vi "Lavatory_System..vi"(11 "Error_In":errorcluster) -> (15 "Error_Out":errorcluster)   [LabVIEW 2021]
doc: "This is the Main VI that performs the Lavatory system."
uses:
  Controls/Lavatory.ctl
  Controls/Lavatory_Data.ctl
  Controls/Queue_Operation_Select.ctl
  Controls/Timer_Operation_Select.ctl
panel:
  in  "Stop_Simulation":bool
  in  "Alarm_Timer_Limit":dbl=2.0 caption="Alarm Timer Limit" min=1.0 max=300.0
  out "Alarm_Timer_D":dbl caption="Alarm Timer D"
  out "Alarm_Timer_C":dbl caption="Alarm Timer C"
  in  "Lavatory_D_Occupied":bool caption="Lavatory D Occupied"
  in  "Lavatory_C_Occupied":bool caption="Lavatory C Occupied"
  out "Alarm_Timer_B":dbl caption="Alarm Timer B"
  out "Alarm_Timer_A":dbl caption="Alarm Timer A"
  in  "Lavatory_B_Occupied":bool caption="Lavatory B Occupied"
  in  "Lavatory_A_Occupied":bool caption="Lavatory A Occupied"
  out "Rear_Lavatories_Occupied":bool caption="Lavatories\nOccupied"
  out "Front_Lavatories_Occupied":bool caption="Lavatories\nOccupied"
  in  "Alarm_Achnowledge":bool caption="Alarm Achnowledge"
  out "Lavatory":string
  out "Alarm":bool
  in  "Seatbelt_Sign_ON":bool caption="Seatbelt Sign ON"
  out "Lavatory_A":T1 caption="Lavatory A"
  out "Lavatory_B":T1 caption="Lavatory B"
  out "Lavatory_D":T1 caption="Lavatory D"
  out "Lavatory_C":T1 caption="Lavatory C"
  # "Airplane Lavatory Signs"
  # "Front"
  # "Rear"
  # "Steward's Area"
  # "Simulation Contols & Indicators"
  # "Secs"
  # "Secs"
  # "Secs"
  # "Secs"
  # "Secs"
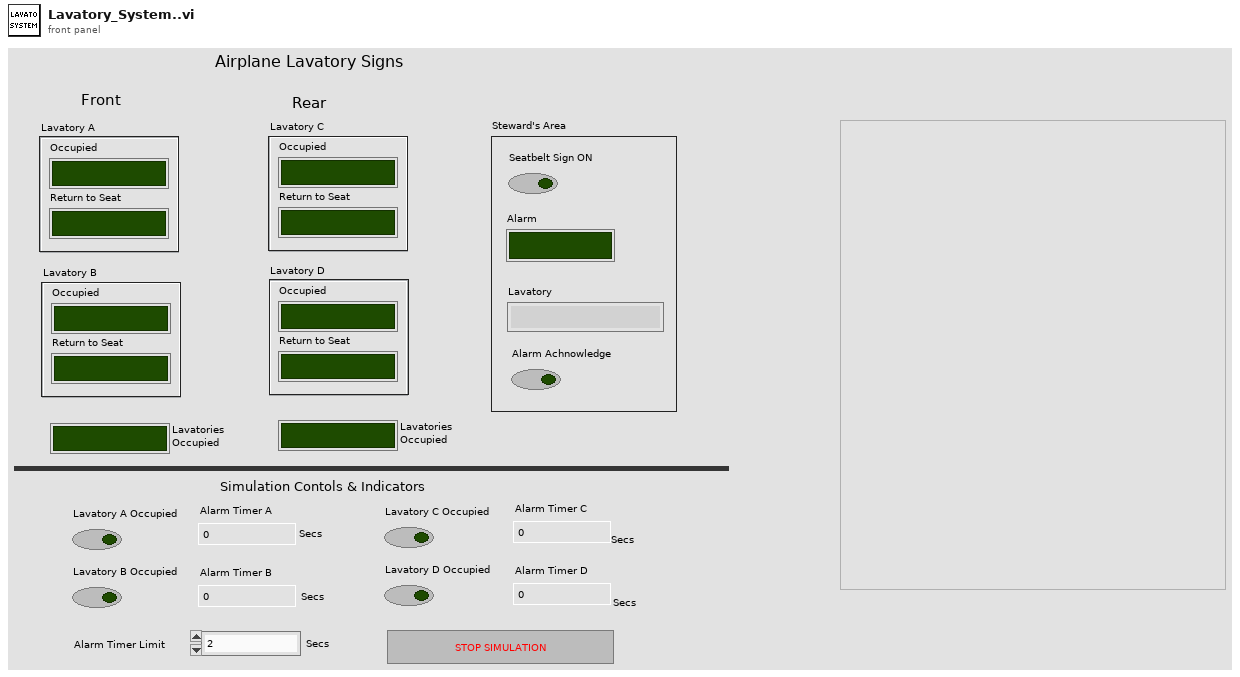
[diagram p1: front panel]
types:
  T1 = typedef "Lavatory.ctl" = cluster{"Occupied":bool, "Return_To_Seat":bool}
  T2 = typedef "Queue_Operation_Select.ctl" = enum16{"Obtain_Queue", "Enqueue", "Enqueue_N", "Enqueue_at_End", "Dequeue", "Flush", "Release_Queue"}
  T3 = typedef "Lavatory_Data.ctl" = cluster{"Lavatory":T1, "Lavatory_Name":string[], "Rear_Lavatories_Occupied":bool, "Front_Lavatories_Occupied":bool, "Alarm_Time":dbl[], "Alarm":bool, "Alarm_Message":string, "Alarm_Timer_Limit":dbl, "Seatbelt_Sign_ON":bool, "Occupied":bool[], "Return_To_Seat_F":bool[], "Lavatory_Reference":refnum<vi>[], "Time_Out?":bool[], "Lavatory_Controls":refnum<vi>[]}
  T4 = typedef "Timer_Operation_Select.ctl" = enum16{"Initialize", "Start_Timer", "Time_Out?", "Stop_Timer"}
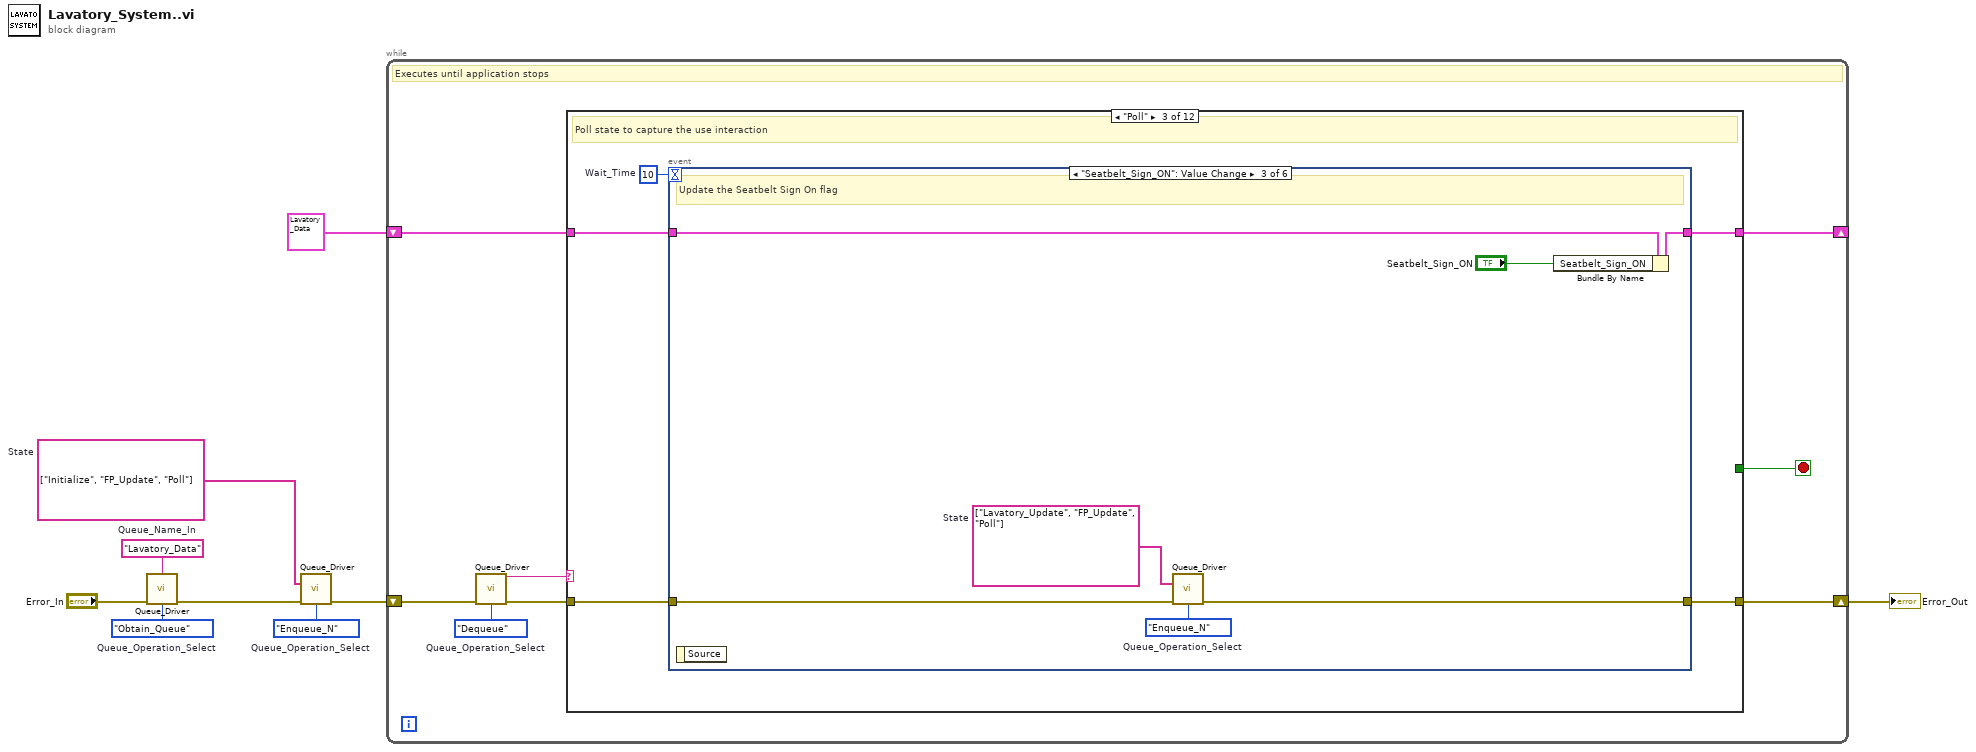
[diagram p0: block diagram]
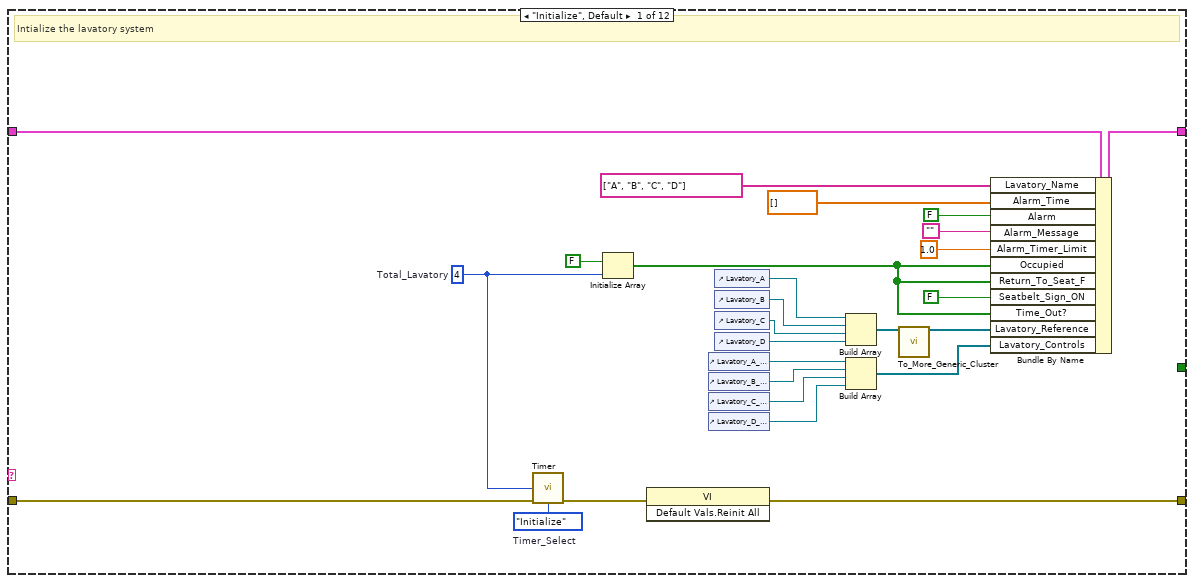
[diagram p2: hidden frame]
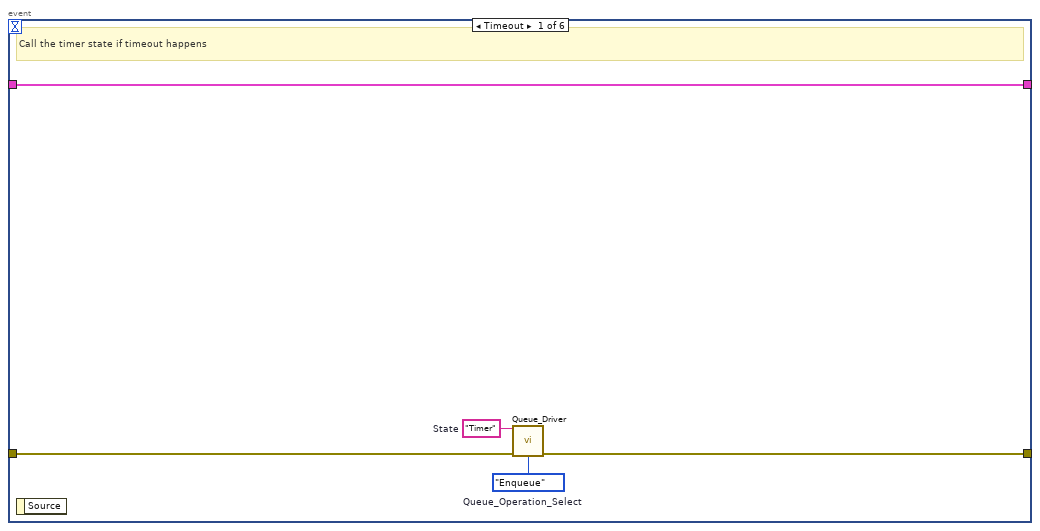
[diagram p4: hidden frame]
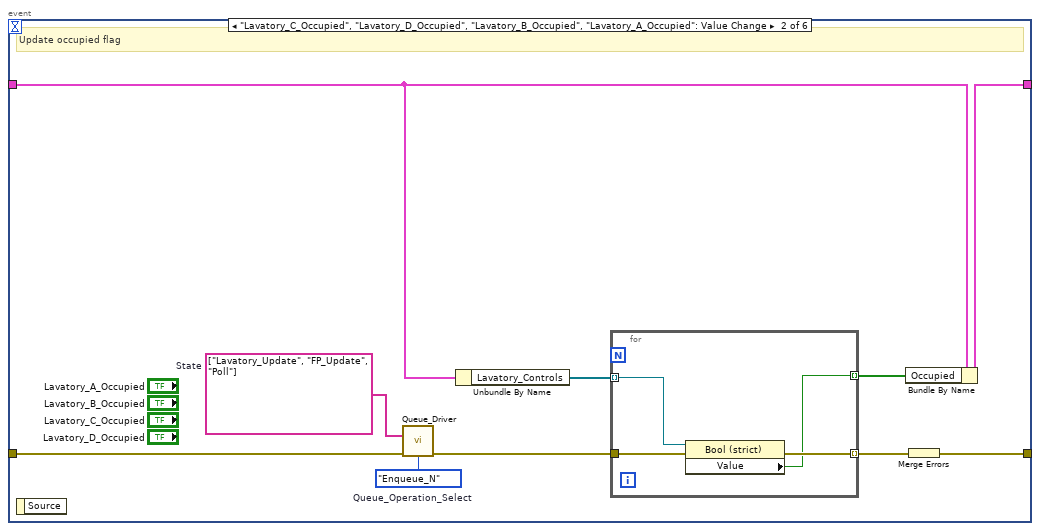
[diagram p5: hidden frame]
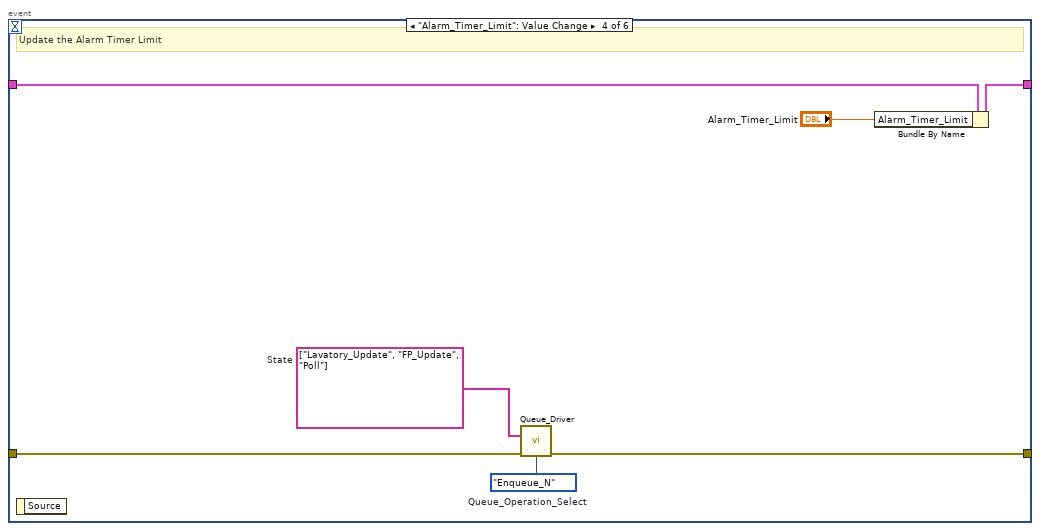
[diagram p6: hidden frame]
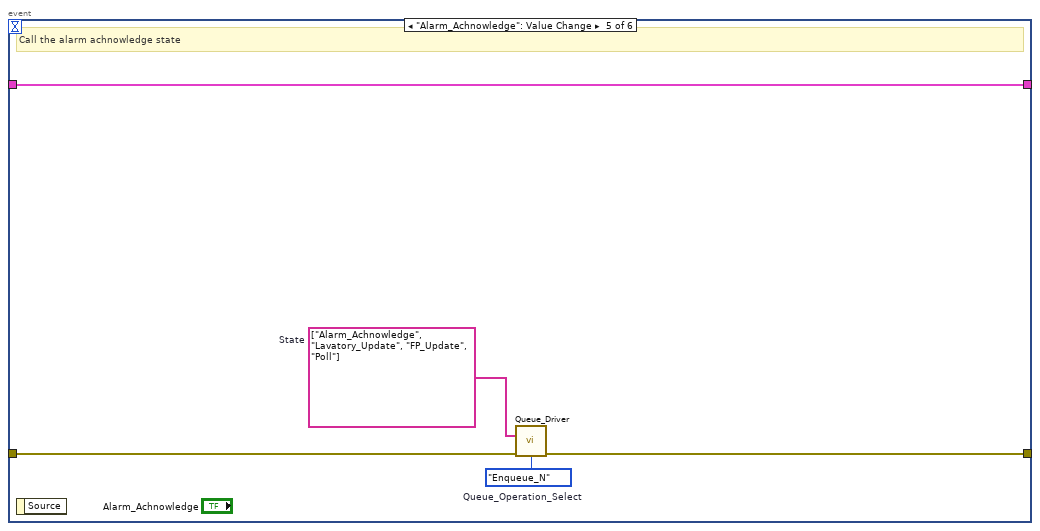
[diagram p7: hidden frame]
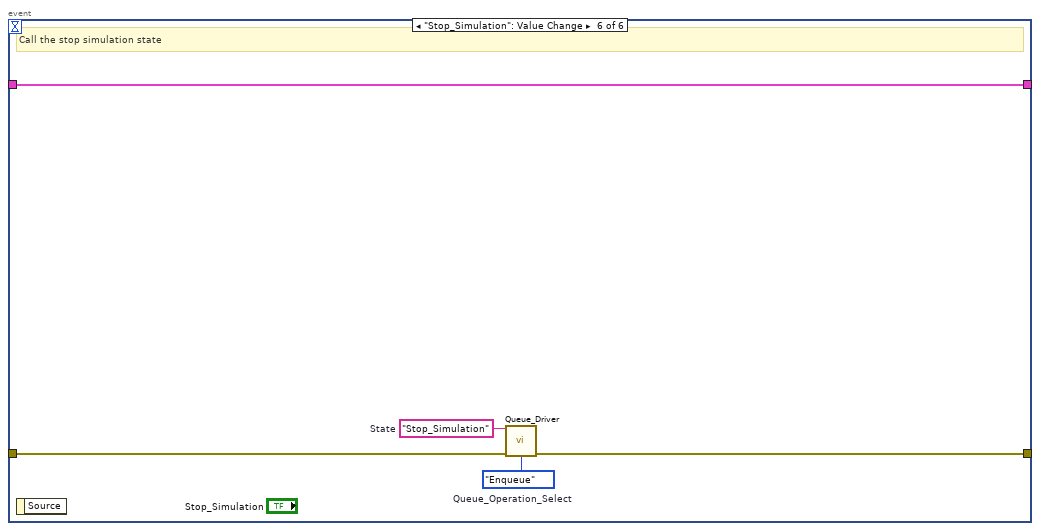
[diagram p8: hidden frame]
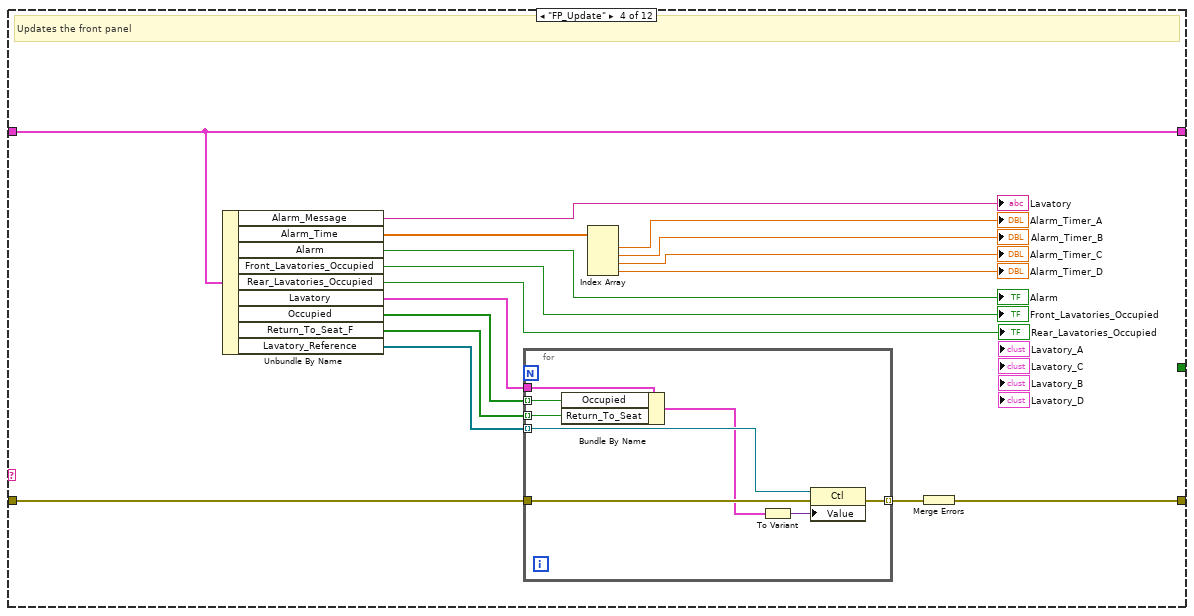
[diagram p9: hidden frame]
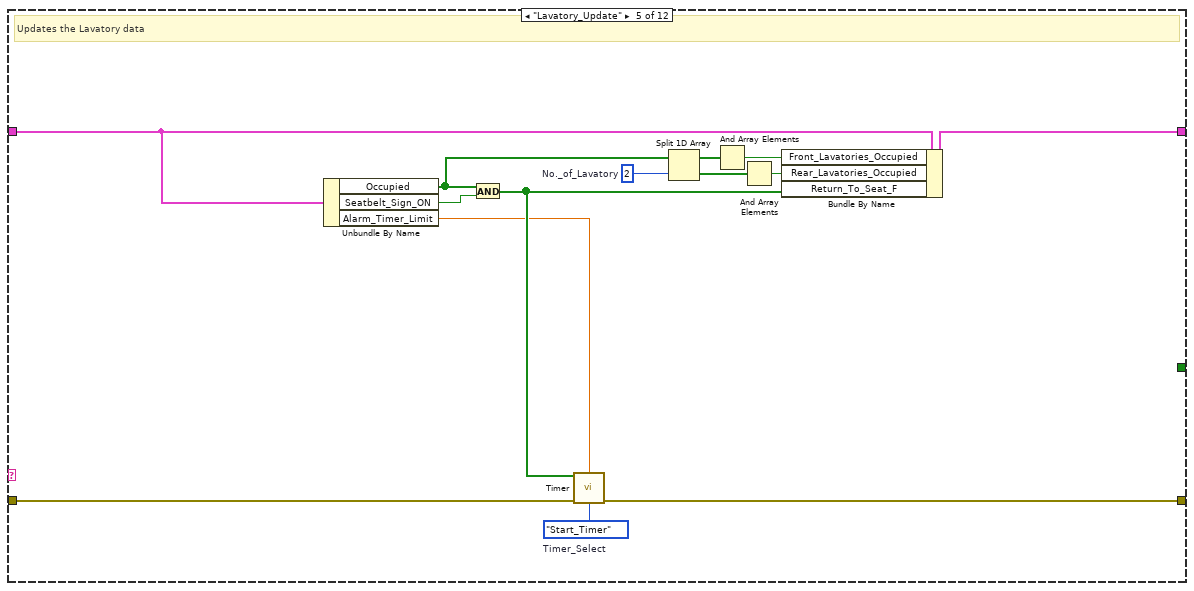
[diagram p10: hidden frame]
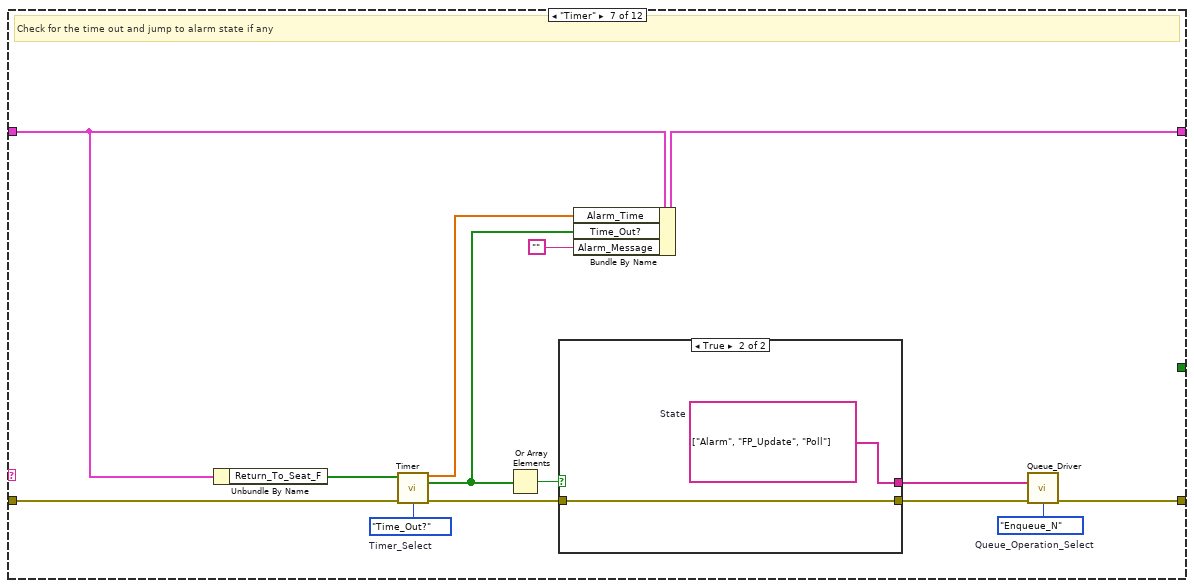
[diagram p12: hidden frame]
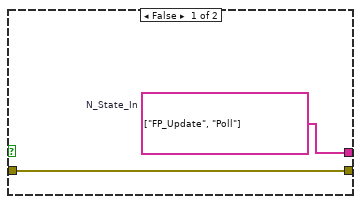
[diagram p13: hidden frame]
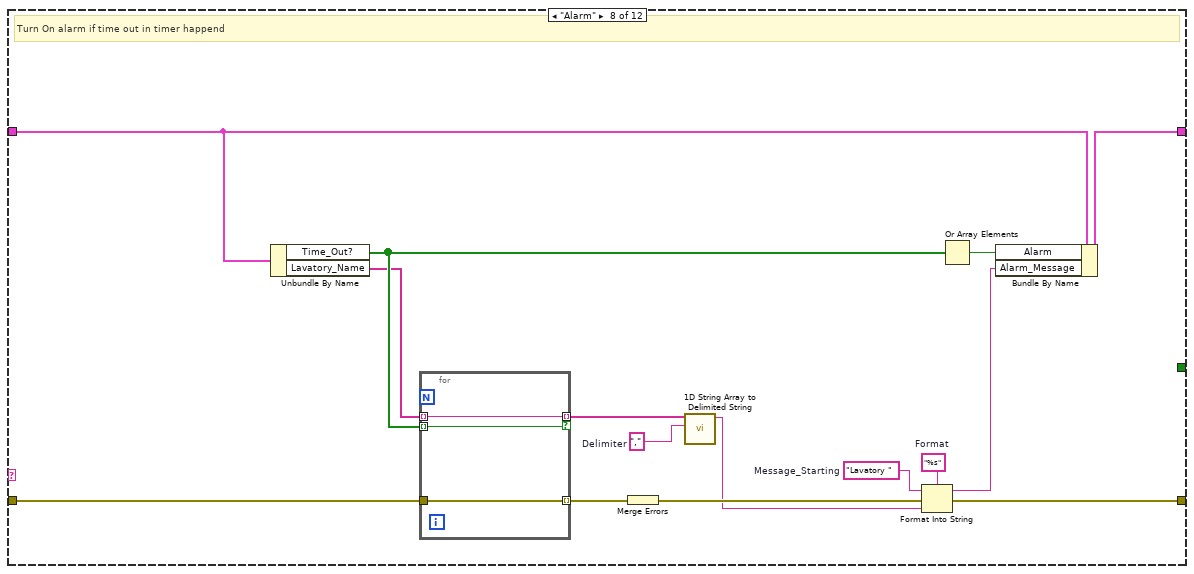
[diagram p14: hidden frame]
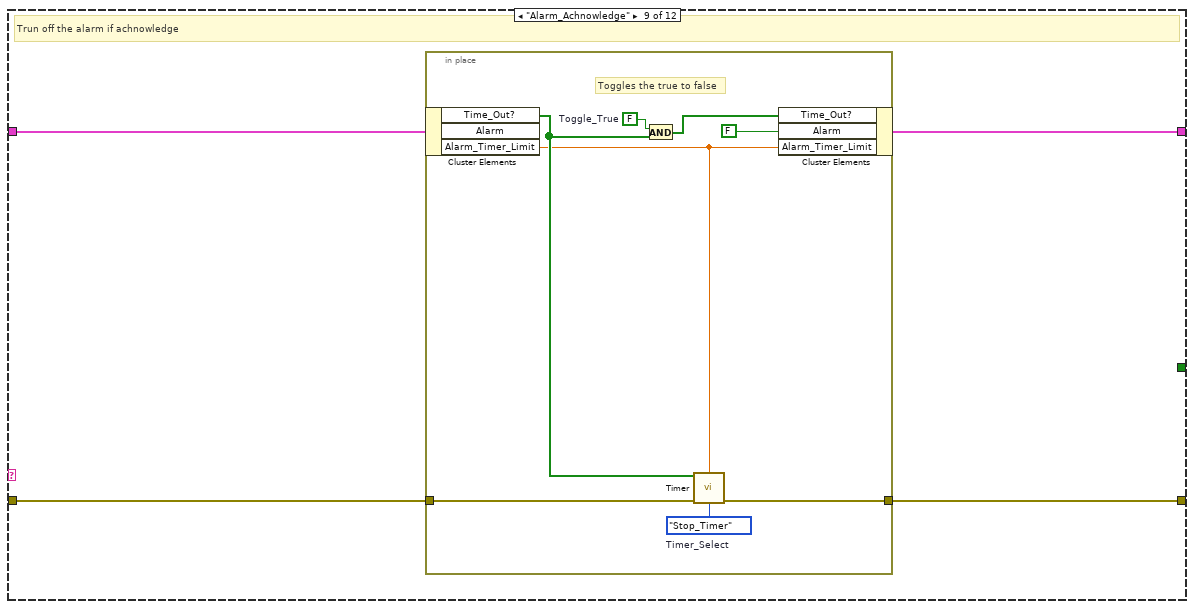
[diagram p15: hidden frame]
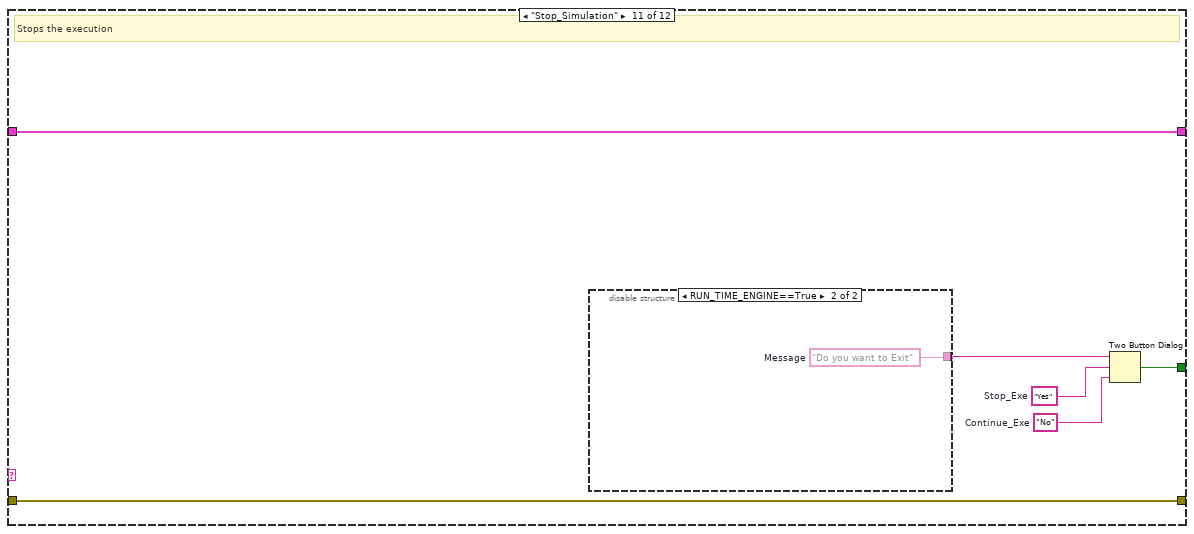
[diagram p17: hidden frame]
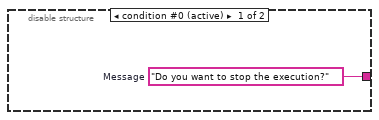
[diagram p18: hidden frame]
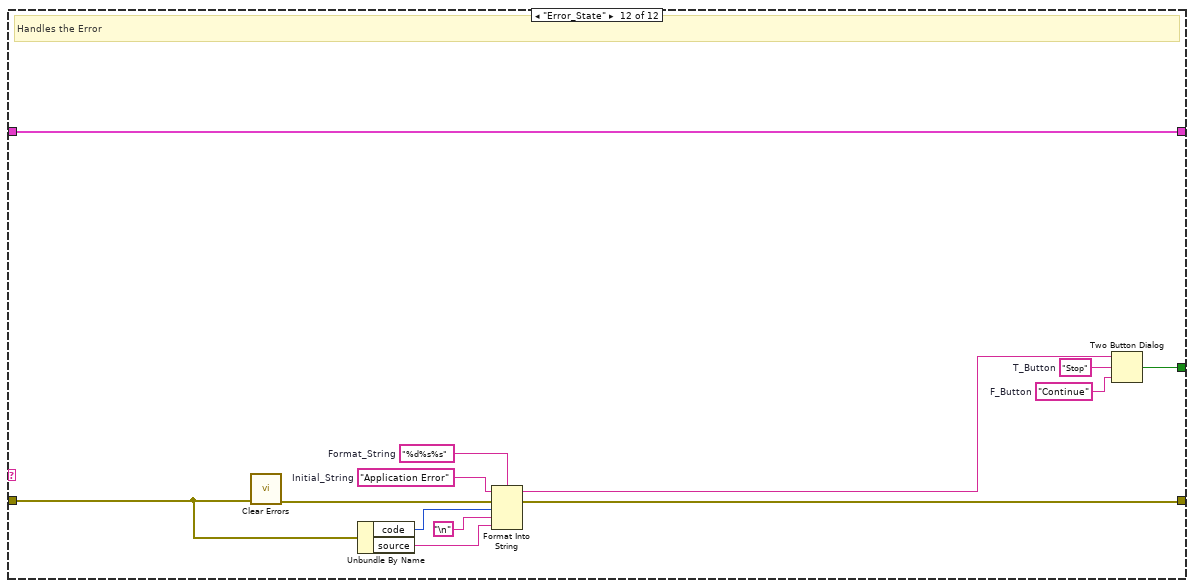
[diagram p19: hidden frame]
diagram:
  w3 = Queue_Operation_Select."Enqueue_N"  # Queue_Operation_Select
  w2 = string[] ["Initialize", "FP_Update", "Poll"]  # State
  w5 = Queue_Operation_Select."Obtain_Queue"  # Queue_Operation_Select
  w6 = "Lavatory_Data"  # Queue_Name_In
  n1 = call "Queue_Driver.vi"("Queue_Name_In"=w6, "Error_In"="Error_In", "Queue_Operation_Select"=w5) -> ("Error_Out"=w7:errorcluster)  [unwired: 11 in, 1 out]
  n2 = call "Queue_Driver.vi"("N_State_In"=w2, "Error_In"=w7, "Queue_Operation_Select"=w3) -> ("Error_Out"=w1:errorcluster)  [unwired: 11 in, 1 out]
  n3 = while {
    shift-right: [w12] -> _
    shift-left: T3 {"Lavatory"={"Occupied"=FALSE, "Return_To_Seat"=FALSE}, "Lavatory_Name"=[], "Rear_Lavatories_Occupied"=FALSE, "Front_Lavatories_Occupied"=FALSE, "Alarm_Time"=[], "Alarm"=FALSE, "Alarm_Message"="", "Alarm_Timer_Limit"=0.0, "Seatbelt_Sign_ON"=FALSE, "Occupied"=[], "Return_To_Seat_F"=[], "Lavatory_Reference"=[], "Time_Out?"=[], "Lavatory_Controls"=[]} -> [w13]
    shift-right: [w17] -> w8
    shift-left: w1 -> [w16]
    stop <- w10 stop-if-true
    w14 = Queue_Operation_Select."Dequeue"  # Queue_Operation_Select
    # "Executes until application stops"
    n4 = call "Queue_Driver.vi"("Error_In"=w16, "Queue_Operation_Select"=w14) -> ("State_Out"=w15:string, "Error_Out"=w11:errorcluster)  [unwired: 12 in]
    n5 = case shown="\"Poll\"" w15 {
      tunnel: [w22 w44 w46 w100 w128 w133 w144 w153 w171 w183 w190 w195] -> w17
      tunnel: w11 -> [w43 w44 w50 w106 w132 w133 w147 w160 w172 w183 w190 w196]
      tunnel: w13 -> [w28 w45 w49 w107 w130 w134 w142 w167 w173 w184 w189 w193]
      tunnel: [w42 w45 w47 w107 w129 w134 w143 w166 w174 w184 w189 w193] -> w12
      tunnel: [_ _ _ _ _ _ _ _ _ _ w187 w194] -> w10
      frame "Initialize", Default {
        w23 = Timer_Operation_Select."Initialize"  # Timer_Select
        w24 = 4  # Total_Lavatory
        # "Intialize the lavatory system"
        n6 = call "Timer.vi"("Timer_Required"=w24, "Error_In"=w43, "Timer_Select"=w23) -> ("Error_Out"=w25:errorcluster)  [unwired: 10 in, 2 out]
        n7 = Initialize Array(FALSE, w24) -> (w27:bool[])
        n8 = invoke class="VI" method="Default Vals.Reinit All"(error in=w25) -> (error out=w22:errorcluster)  [unwired: 2 in, 2 out]
        n9 = control-ref of="Lavatory_A_Occupied"() -> (w32:refnum<vi>)
        n10 = control-ref of="Lavatory_B_Occupied"() -> (w31:refnum<vi>)
        n11 = control-ref of="Lavatory_C_Occupied"() -> (w30:refnum<vi>)
        n12 = control-ref of="Lavatory_D_Occupied"() -> (w29:refnum<vi>)
        n13 = control-ref of="Lavatory_A"() -> (w40:refnum<vi>)
        n14 = control-ref of="Lavatory_B"() -> (w39:refnum<vi>)
        n15 = control-ref of="Lavatory_C"() -> (w38:refnum<vi>)
        n16 = control-ref of="Lavatory_D"() -> (w37:refnum<vi>)
        n17 = Build Array(w40, w39, w38, w37) -> (w19:refnum<vi>[])
        n18 = Build Array(w32, w31, w30, w29) -> (w20:refnum<vi>[])
        n19 = call "To_More_Generic_Cluster.vi"("Reference_In"=w19) -> ("Reference_Out"=w18:refnum<vi>[])  [unwired: 14 in]
        n20 = Bundle By Name(cluster=w28, "Lavatory_Name"=string[] ["A", "B", "C", "D"], "Alarm_Time"=dbl[] [] ("Alarm_Timer_A"), "Alarm"=FALSE ("Stop_Simulation"), "Alarm_Message"="" ("Lavatory"), "Alarm_Timer_Limit"=1.0, "Occupied"=w27, "Return_To_Seat_F"=w27, "Seatbelt_Sign_ON"=FALSE, "Time_Out?"=w27, "Lavatory_Reference"=w18, "Lavatory_Controls"=w20) -> (w42:T3)
      }
      frame "------------------Update_Users----------------" {
        # "States after this are caused due to user interaction"
      }
      frame "Poll" {
        w48 = 10  # Wait_Time
        # "Poll state to capture the use interaction"
        n21 = event shown="[2] \"Seatbelt_Sign_ON\": Value Change" {
          selector: _ -> [_ _ _ _ _ _]
          dyn-events: _ -> [_ _ _ _ _ _]
          timeout: w48 -> [_ _ _ _ _ _]
          tunnel: [w54 w59 w75 w79 w86 w91] -> w46
          tunnel: w50 -> [w55 w65 w76 w81 w87 w92]
          tunnel: w49 -> [w51 w56 w73 w83 w88 w93]
          tunnel: [w51 w64 w72 w82 w88 w93] -> w47
          event Timeout {
            w52 = "Timer"  # State
            w53 = Queue_Operation_Select."Enqueue"  # Queue_Operation_Select
            # "Call the timer state if timeout happens"
            n22 = event-data() -> ()  [unwired: 1 in, 1 out]
            n23 = call "Queue_Driver.vi"("State_In"=w52, "Error_In"=w55, "Queue_Operation_Select"=w53) -> ("Error_Out"=w54:errorcluster)  [unwired: 11 in, 1 out]
          }
          event "Lavatory_C_Occupied", "Lavatory_D_Occupied", "Lavatory_B_Occupied", "Lavatory_A_Occupied": Value Change {
            w61 = string[] ["Lavatory_Update", "FP_Update", "Poll"]  # State
            w62 = Queue_Operation_Select."Enqueue_N"  # Queue_Operation_Select
            # "Update occupied flag"
            n24 = event-data() -> ()  [unwired: 1 in, 1 out]
            n25 = call "Queue_Driver.vi"("N_State_In"=w61, "Error_In"=w65, "Queue_Operation_Select"=w62) -> ("Error_Out"=w63:errorcluster)  [unwired: 11 in, 1 out]
            n26 = Unbundle By Name(w56) -> ("Lavatory_Controls"=w58:refnum<vi>[])
            n27 = for {
              tunnel: w63 -> [w69]
              tunnel: [w67] -> w60 mode=indexing
              tunnel: w58 -> [w68] mode=indexing
              tunnel: [w66] -> w57 mode=indexing
              n28 = property class="Bool (strict)"(reference=w68, error in=w69) -> (error out=w67:errorcluster, "Value"=w66:bool)  [unwired: 1 out]
            }
            n29 = Bundle By Name(cluster=w56, "Occupied"=w57) -> (w64:T3)
            n30 = Merge Errors(w60) -> (w59:errorcluster)
          }
          event "Seatbelt_Sign_ON": Value Change {
            w70 = string[] ["Lavatory_Update", "FP_Update", "Poll"]  # State
            w74 = Queue_Operation_Select."Enqueue_N"  # Queue_Operation_Select
            # "Update the Seatbelt Sign On flag"
            n31 = event-data() -> ()  [unwired: 1 in, 1 out]
            n32 = call "Queue_Driver.vi"("N_State_In"=w70, "Error_In"=w76, "Queue_Operation_Select"=w74) -> ("Error_Out"=w75:errorcluster)  [unwired: 11 in, 1 out]
            n33 = Bundle By Name(cluster=w73, "Seatbelt_Sign_ON"="Seatbelt_Sign_ON") -> (w72:T3)
          }
          event "Alarm_Timer_Limit": Value Change {
            w77 = string[] ["Lavatory_Update", "FP_Update", "Poll"]  # State
            w78 = Queue_Operation_Select."Enqueue_N"  # Queue_Operation_Select
            # "Update the Alarm Timer Limit"
            n34 = event-data() -> ()  [unwired: 1 in, 1 out]
            n35 = call "Queue_Driver.vi"("N_State_In"=w77, "Error_In"=w81, "Queue_Operation_Select"=w78) -> ("Error_Out"=w79:errorcluster)  [unwired: 11 in, 1 out]
            n36 = Bundle By Name(cluster=w83, "Alarm_Timer_Limit"="Alarm_Timer_Limit") -> (w82:T3)
          }
          event "Alarm_Achnowledge": Value Change {
            w84 = string[] ["Alarm_Achnowledge", "Lavatory_Update", "FP_Update", "Poll"]  # State
            w85 = Queue_Operation_Select."Enqueue_N"  # Queue_Operation_Select
            # "Call the alarm achnowledge state"
            n37 = event-data() -> ()  [unwired: 1 in, 1 out]
            n38 = call "Queue_Driver.vi"("N_State_In"=w84, "Error_In"=w87, "Queue_Operation_Select"=w85) -> ("Error_Out"=w86:errorcluster)  [unwired: 11 in, 1 out]
          }
          event "Stop_Simulation": Value Change {
            w89 = Queue_Operation_Select."Enqueue"  # Queue_Operation_Select
            w90 = "Stop_Simulation"  # State
            # "Call the stop simulation state"
            n39 = event-data() -> ()  [unwired: 1 in, 1 out]
            n40 = call "Queue_Driver.vi"("State_In"=w90, "Error_In"=w92, "Queue_Operation_Select"=w89) -> ("Error_Out"=w91:errorcluster)  [unwired: 11 in, 1 out]
          }
        }
      }
      frame "FP_Update" {
        # "Updates the front panel"
        n41 = Unbundle By Name(w107) -> ("Alarm_Message"=→"Lavatory":string, "Alarm_Time"=w98:dbl[], "Alarm"=→"Alarm":bool, "Front_Lavatories_Occupied"=→"Front_Lavatories_Occupied":bool, "Rear_Lavatories_Occupied"=→"Rear_Lavatories_Occupied":bool, "Lavatory"=w102:T1, "Occupied"=w104:bool[], "Return_To_Seat_F"=w103:bool[], "Lavatory_Reference"=w101:refnum<vi>[])
        n42 = for {
          tunnel: w101 -> [w113] mode=indexing
          tunnel: w104 -> [w117] mode=indexing
          tunnel: w103 -> [w118] mode=indexing
          tunnel: w102 -> [w116]
          tunnel: w106 -> [w115]
          tunnel: [w114] -> w105 mode=indexing
          n43 = Bundle By Name(cluster=w116, "Occupied"=w117, "Return_To_Seat"=w118) -> (w112:T1)
          n44 = To Variant(anything=w112) -> (Variant=w111:variant)
          n45 = property class="Ctl"(reference=w113, error in=w115, "Value"=w111) -> (error out=w114:errorcluster)  [unwired: 1 out]
        }
        n46 = Index Array(array=w98) -> (element #1=→"Alarm_Timer_A":dbl, element #2=→"Alarm_Timer_B":dbl, element #3=→"Alarm_Timer_C":dbl, element #4=→"Alarm_Timer_D":dbl)  [unwired: 4 in]
        n47 = Merge Errors(w105) -> (w100:errorcluster)
      }
      frame "Lavatory_Update" {
        w122 = 2  # No._of_Lavatory
        w131 = Timer_Operation_Select."Start_Timer"  # Timer_Select
        # "Updates the Lavatory data"
        n48 = Unbundle By Name(w130) -> ("Occupied"=w120:bool[], "Seatbelt_Sign_ON"=w121:bool, "Alarm_Timer_Limit"=w119:dbl)
        n49 = And(x=w120, y=w121) -> (x .and. y?=w127:bool[])
        n50 = call "Timer.vi"("Timers_Start"=w127, "Wait_Time"=w119, "Error_In"=w132, "Timer_Select"=w131) -> ("Error_Out"=w128:errorcluster)  [unwired: 9 in, 2 out]
        n51 = Split 1D Array(array=w120, index=w122) -> (first subarray=w126:bool[], second subarray=w124:bool[])
        n52 = And Array Elements(Boolean array=w126) -> (logical AND=w125:bool)
        n53 = And Array Elements(Boolean array=w124) -> (logical AND=w123:bool)
        n54 = Bundle By Name(cluster=w130, "Front_Lavatories_Occupied"=w125, "Rear_Lavatories_Occupied"=w123, "Return_To_Seat_F"=w127) -> (w129:T3)
      }
      frame "-----------------Timer_and_Alarm-------------" {
        # "States after this are timer and alarm related states"
      }
      frame "Timer" {
        w145 = Queue_Operation_Select."Enqueue_N"  # Queue_Operation_Select
        w148 = Timer_Operation_Select."Time_Out?"  # Timer_Select
        # "Check for the time out and jump to alarm state if any"
        n55 = Unbundle By Name(w142) -> ("Return_To_Seat_F"=w141:bool[])
        n56 = call "Timer.vi"("Timers_Start"=w141, "Error_In"=w147, "Timer_Select"=w148) -> ("Timer_Time"=w139:dbl[], "Time_Out?"=w135:bool[], "Error_Out"=w137:errorcluster)  [unwired: 10 in]
        n57 = Or Array Elements(Boolean array=w135) -> (logical OR=w136:bool)
        n58 = case shown="True" w136 {
          tunnel: [w149 w152] -> w146
          tunnel: [w150 w151] -> w138
          tunnel: w137 -> [w150 w151]
          frame False {
            w149 = string[] ["FP_Update", "Poll"]  # N_State_In
          }
          frame True {
            w152 = string[] ["Alarm", "FP_Update", "Poll"]  # State
          }
        }
        n59 = Bundle By Name(cluster=w142, "Alarm_Time"=w139, "Time_Out?"=w135, "Alarm_Message"="" ("Lavatory")) -> (w143:T3)
        n60 = call "Queue_Driver.vi"("N_State_In"=w146, "Error_In"=w138, "Queue_Operation_Select"=w145) -> ("Error_Out"=w144:errorcluster)  [unwired: 11 in, 1 out]
      }
      frame "Alarm" {
        w156 = ","  # Delimiter
        w163 = "%s"  # Format
        w162 = "Lavatory "  # Message_Starting
        # "Turn On alarm if time out in timer happend"
        n61 = Unbundle By Name(w167) -> ("Time_Out?"=w164:bool[], "Lavatory_Name"=w154:string[])
        n62 = for {
          tunnel: w164 -> [w168] mode=indexing
          tunnel: w154 -> [w169] mode=indexing
          tunnel: w160 -> [w170]
          tunnel: [w170] -> w159 mode=indexing
          tunnel: [w169] -> w157 mode=indexing if=w168
        }
        n63 = Merge Errors(w159) -> (w158:errorcluster)
        n64 = call <vilib>:"1D String Array to Delimited String.vi"("delimiter"=w156, "string array"=w157) -> ("delimited string"=w155:string)  [unwired: 9 in]
        n65 = Format Into String(format string=w163, initial string=w162, error in=w158, w155) -> (resulting string=w161:string, error out=w153:errorcluster)
        n66 = Or Array Elements(Boolean array=w164) -> (logical OR=w165:bool)
        n67 = Bundle By Name(cluster=w167, "Alarm"=w165, "Alarm_Message"=w161) -> (w166:T3)
      }
      frame "Alarm_Achnowledge" {
        # "Trun off the alarm if achnowledge"
        n68 = in-place "In Place Element Structure" {
          in-place-border: w172 -> [w182]
          in-place-border: [w181] -> w171
          w180 = Timer_Operation_Select."Stop_Timer"  # Timer_Select
          w177 = FALSE  # Toggle_True
          # "Toggles the true to false"
          n69 = in-place-cluster #1(w173) -> ("Time_Out?"=w176:bool[], "Alarm_Timer_Limit"=w175:dbl)  [unwired: 1 out]
          n70 = And(x=w177, y=w176) -> (x .and. y?=w178:bool[])
          n71 = call "Timer.vi"("Timers_Start"=w176, "Wait_Time"=w175, "Error_In"=w182, "Timer_Select"=w180) -> ("Error_Out"=w181:errorcluster)  [unwired: 9 in, 2 out]
          n72 = in-place-cluster #1("Time_Out?"=w178, "Alarm"=FALSE, "Alarm_Timer_Limit"=w175) -> (w174:T3)
        }
      }
      frame "----------------------- Exit---------------------" {
        # "States after this are exit related"
      }
      frame "Stop_Simulation" {
        w186 = "No"  # Continue_Exe
        w185 = "Yes"  # Stop_Exe
        # "Stops the execution"
        n73 = disable-structure "Conditional Disable Structure" shown="RUN_TIME_ENGINE==True" {
          disable-tunnel: [w191 w192] -> w188
          frame condition #0 (active) {
            w191 = "Do you want to stop the execution?"  # Message
          }
          frame condition #1 {
            w192 = "Do you want to Exit"  # Message
          }
        }
        n74 = Two Button Dialog(message=w188, 1:w186, 2:w185) -> (T button?=w187:bool)
      }
      frame "Error_State" {
        w201 = "%d%s%s"  # Format_String
        w202 = "Application Error"  # Initial_String
        w203 = "Stop"  # T_Button
        w204 = "Continue"  # F_Button
        # "Handles the Error"
        n75 = call <vilib>:"Clear Errors.vi"("error in (no error)"=w196) -> ("error out"=w199:errorcluster)  [unwired: 5 in, 1 out]
        n76 = Unbundle By Name(w196) -> ("code"=w198:i32, "source"=w197:string)
        n77 = Format Into String(format string=w201, initial string=w202, error in=w199, w198, "\n" ("Line Feed Constant"), w197) -> (resulting string=w205:string, error out=w195:errorcluster)
        n78 = Two Button Dialog(message=w205, 1:w204, 2:w203) -> (T button?=w194:bool)
      }
    }
  }
  "Error_Out" <- w8
